vi "NF87XX.enable closed loop mode.vi"(0 "i ref in":refnum<vi>, 2 "Enable closed loop mode":bool, 5 "error in (no error)":errorcluster) -> (14 "i ref out":refnum<vi>, 19 "error out":errorcluster)   [LabVIEW 2014, in "NF87XX.lvlib"]
doc: "Turns on/off the closed loop mode of the driver (only valid when used with the model 8751-C closed loop driver). \n\nauthor: Stefan Götte\ndata: 09-JAN-2007\n\n\nLicense Agreement for this software:\n\nCopyright (C)\nGesellschaft für Schwerionenforschung, GSI\nPlanckstr. 1\n64291 Darmstadt\nGermany\n\nContact: D.Beck@gsi.de \n\nThis program is free software; you can redistribute it and/or modify it under the terms of the GNU General Public License as published by the Free Software Foundation; either version 2 of the license, or (at your option) any later version.\n\nThis program is distributed in the hope that it will be useful, but WITHOUT ANY WARRANTY; without even the implied warranty of MERCHANTABILITY or FITNESS FOR A PARTICULAR PURPOSE. See the GNU General License for more details (http://www.gnu.org).\n\nGesellschaft für Schwerionenforschung, GSI\nPlanckstr. 1, 64291 Darmstadt, Germany\nFor all questions and ideas contact: M.Richter@gsi.de, H.Brand@gsi.de or D.Beck@gsi.de.\nLast update: 17-JUN-2004"
uses:
  NF87XX.lvlib
  instr.lib/NewFocusPico/Pico Parameters.ctl
  instr.lib/NewFocusPico/NewFocusPico - Driver np.lvlib
panel:
  in  "System":string="N/A"
  in  "Pico Parameter type":T1={"Pico Type"=enum."Open-Loop Pico", "Acceleration (steps/sec^2)"="32000", "Velocity ( Hz)"="2000", "Driver"="A1", "Motor"="0", "Channel"="0", "Process Step"="Final Test"}
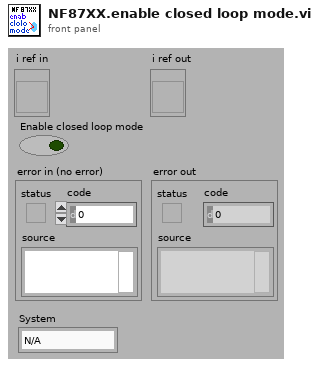
[diagram p1: front panel]
types:
  T1 = typedef "NewFocusPico - Driver np.lvlib/Pico Parameters.ctl" = cluster{"Pico Type":enum16{"Open-Loop Pico", "Close-Loop Pico", "Pico Ultra"}, "Acceleration (steps/sec^2)":string, "Velocity ( Hz)":string, "Driver":string, "Motor":string, "Channel":string, "Process Step":string}
  T2 = typedef "NF87XX.lvlib/NF87XX.driver Type.ctl" = enum16{"not defined", "3-ch open loop drv", "1-ch closed loop drv"}
  T3 = enum16{"User....", "DEF", "DIAG", "INI", "LOCK", "UNLOCK", "MAP", "SAV", "VER", "ACC", "CHL", "FOR", "GO", "HAL", "MOF", "MON", "MPV", "POS", "REL", "REV", "STA", "STO", "TYP", "VEL", "ABS", "SER", "NOS", "DRT", "FLI", "RLI", "FIN", "RIN", "AIN", "IN", "JOF", "JON", "OUT", "RES FINE", "RES COARSE", "02 (HEX)", "PWM", "CNT", "TMR", "HOSTNAME", "IPADDR", "IPMODE", "NETMASK", "GATEWAY", "DNSSRVR", "PASSWD", "ECHO", "MACADDR"}
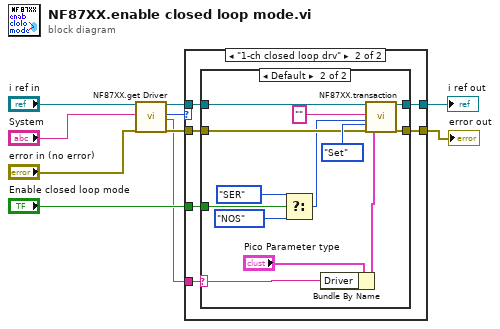
[diagram p0: block diagram]
diagram:
  n1 = call "NF87XX.get Driver.vi"("i ref in"="i ref in", "System"="System", "error in (no error)"="error in (no error)") -> ("i ref out"=w5:refnum<vi>, "Driver Type"=w1:T2, "Driver"=w2:string, "error out"=w6:errorcluster)  [unwired: 12 in, 1 out]
  n2 = case shown="\"1-ch closed loop drv\"" w1 {
    tunnel: [w12 w18] -> w10
    tunnel: [w11 w17] -> w9
    tunnel: w6 -> [w11 w16]
    tunnel: w5 -> [w12 w15]
    tunnel: "Enable closed loop mode" -> [_ w14]
    tunnel: w2 -> [_ w13]
    frame "not defined", Default {
    }
    frame "1-ch closed loop drv" {
      n3 = case shown="Default" w13 {
        selector: w13 -> [_ w21]
        tunnel: [w20 w33] -> w18
        tunnel: [w19 w32] -> w17
        tunnel: w16 -> [w19 w29]
        tunnel: w15 -> [w20 w28]
        tunnel: w14 -> [_ w25]
        frame "N/A" {
        }
        frame Default {
          n4 = Select(t=T3."SER" ("MCL Cmd"), s=w25, f=T3."NOS" ("MCL Cmd")) -> (s? t:f=w22:T3)
          n5 = Bundle By Name(cluster="Pico Parameter type", "Driver"=w21) -> (w26:T1)
          n6 = call "NF87XX.transaction.vi"("i ref in"=w28, "User Cmd/Numeric Argu"="", "MCL Cmd"=w22, "Query/Set"=enum16{"Query", "Set"}."Set", "error in (no error)"=w29, "Pico Parameter"=w26) -> ("i ref out"=w33:refnum<vi>, "error out"=w32:errorcluster)  [unwired: 11 in, 1 out]
        }
      }
    }
  }
  "error out" <- w9
  "i ref out" <- w10
